vi "Send Subscribe.vi"(8 "error in (no error)":errorcluster, 9 "Message ID":u16=10 format="%x", 10 "Subscription Info Array":T1(array[cluster]), 11 "connection ID":refnum<k5>) -> (0 "error out":errorcluster, 3 "connection ID out":refnum<k5>)   [LabVIEW 2020, in "DAQIO MQTT.lvlib"]
doc: "This VI subscribes the client to a selected topic. The client now can read published messages for the topic. \n\n© 2015 - daq.io, LLC - Peter Adelhardt"
uses:
  DAQIO MQTT.lvlib
  Controls/MessageType.ctl
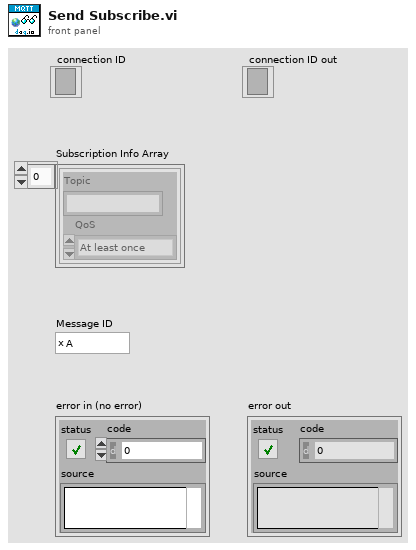
[diagram p1: front panel]
types:
  T1 = cluster{"Topic":string, "QoS":enum8{"At most once", "At least once", "Exactly once", "Reserved"}}[]
  T2 = typedef "DAQIO MQTT.lvlib/MessageType.ctl" = enum32{"Reserved", "CONNECT", "CONNACK", "PUBLISH", "PUBACK", "PUBREC", "PUBREL", "PUBCOMP", "SUBSCRIBE", "SUBACK", "UNSUBSCRIBE", "UNSUBACK", "PINGREQ", "PINGRESP", "DISCONNECT", "Reserved2"}
  T3 = enum8{"At most once", "At least once", "Exactly once", "Reserved"}
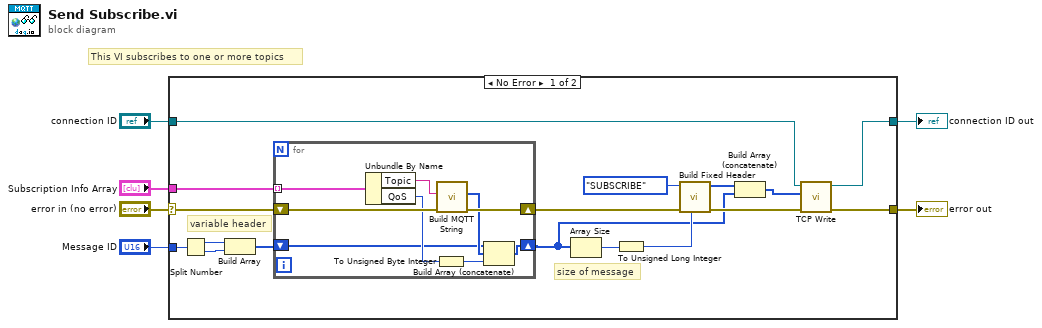
[diagram p0: block diagram]
diagram:
  # "This VI subscribes to one or more topics"
  n1 = case shown="No Error" "error in (no error)" {
    selector: "error in (no error)" -> [w17 w34]
    tunnel: [w12 w34] -> w5
    tunnel: "Message ID" -> [w10 _]
    tunnel: "Subscription Info Array" -> [w9 _]
    tunnel: "connection ID" -> [w8 w33]
    tunnel: [w7 w33] -> w2
    frame No Error {
      # "variable header"
      # "size of message"
      n2 = Split Number(x=w10) -> (hi(x)=w19:u8, lo(x)=w18:u8)
      n3 = Build Array(w19, w18) -> (w16:u8[])
      n4 = for {
        tunnel: w9 -> [w32] mode=indexing
        shift-right: [w29] -> w15
        shift-left: w17 -> [w30]
        shift-right: [w25] -> w11
        shift-left: w16 -> [w24]
        n5 = Unbundle By Name(w32) -> ("Topic"=w31:string, "QoS"=w28:T3)
        n6 = To Unsigned Byte Integer(number=w28) -> (unsigned 8bit integer=w26:u8)
        n7 = call "Build MQTT String.vi"("error in (no error)"=w30, "String to be encoded"=w31) -> ("error out"=w29:errorcluster, "UTF8 Byte Array"=w27:u8[])  [unwired: 8 in]
        n8 = Build Array (concatenate)(w24, w27, w26) -> (w25:u8[])
      }
      n9 = Array Size(array=w11) -> (size(s)=w21:i32)
      n10 = To Unsigned Long Integer(number=w21) -> (unsigned 32bit integer=w22:u32)
      n11 = call "Build Fixed Header.vi"("Remaining Length"=w22, "error in (no error)"=w15, "MessageType"=MessageType."SUBSCRIBE") -> ("error out"=w13:errorcluster, "Fixed Header"=w20:u8[])  [unwired: 7 in]
      n12 = Build Array (concatenate)(w20, w11) -> (w14:u8[])
      n13 = call "TCP Write.vi"("error in (no error)"=w13, "data in"=w14, "connection ID"=w8) -> ("error out"=w12:errorcluster, "connection ID out"=w7:refnum<k5>)  [unwired: 6 in, 1 out]
    }
    frame Error {
    }
  }
  "error out" <- w5
  "connection ID out" <- w2
